vi "Get Picture.vi"(8 "error in (no error)":errorcluster, 11 "Simple Circuit in":refnum<class "Simple Circuit.lvclass">) -> (0 "error out":errorcluster, 2 "Picture":picture, 3 "Simple Circuit out":refnum<class "Simple Circuit.lvclass">)   [LabVIEW 2020, in "Simple Circuit.lvclass"]
uses:
  Simple Circuit.lvclass
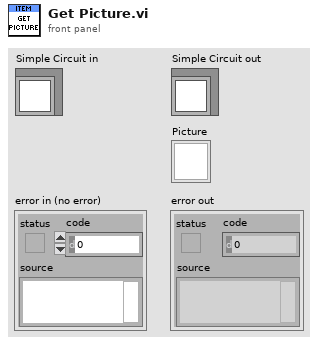
[diagram p1: front panel]
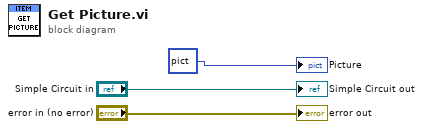
[diagram p0: block diagram]
diagram:
  "error out" <- "error in (no error)"
  "Simple Circuit out" <- "Simple Circuit in"
  "Picture" <- picture bytes[3230] ("new picture")
